vi "Measure AirMar150WX.vi"(8 "error in (no error)":errorcluster, 11 "AirMar150WX in":refnum<class "AirMar150WX.lvclass">) -> (0 "error out":errorcluster, 3 "AirMar150WX out":refnum<class "AirMar150WX.lvclass">)   [LabVIEW 2017, in "AirMar 150WX.lvlib" / "AirMar150WX.lvclass"]
uses:
  AirMar150WX.lvclass
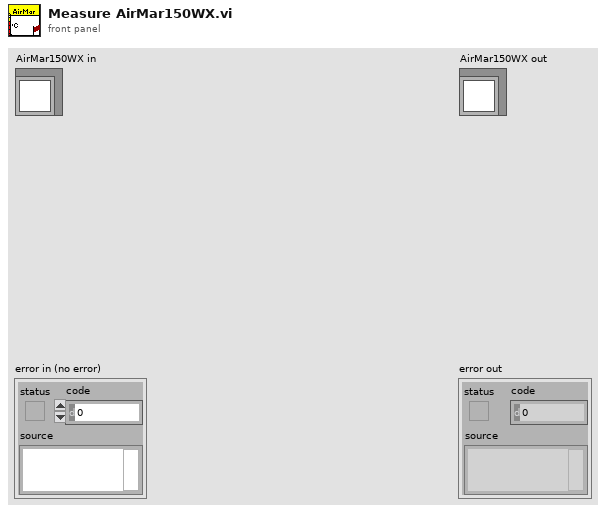
[diagram p1: front panel]
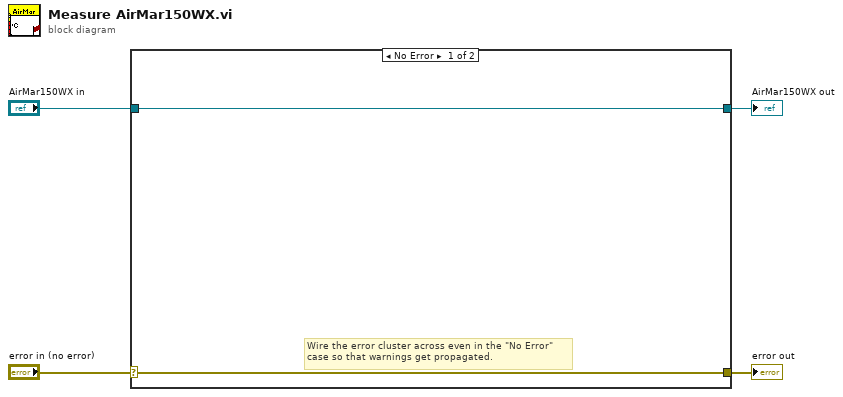
[diagram p0: block diagram]
diagram:
  n1 = case shown="No Error" "error in (no error)" {
    selector: "error in (no error)" -> [w5 w8]
    tunnel: [w5 w8] -> w3
    tunnel: [w6 w7] -> w1
    tunnel: "AirMar150WX in" -> [w6 w7]
    frame No Error {
      # "Wire the error cluster across even in the \"No Error\"\ncase so that warnings get propagated."
    }
    frame Error {
    }
  }
  "error out" <- w3
  "AirMar150WX out" <- w1
